vi "TEST - LVOOP Is Same Or Descendant Class.vi"(8 "error in (no error)":errorcluster) -> (0 "error out":errorcluster, 2 "Pass":bool)   [LabVIEW 2013]
uses:
  LVOOP Data/Class 2/Class 2.lvclass
  LVOOP Data/Class 3/Class 3.lvclass
  LVOOP Data/Class 1/Class 1.lvclass
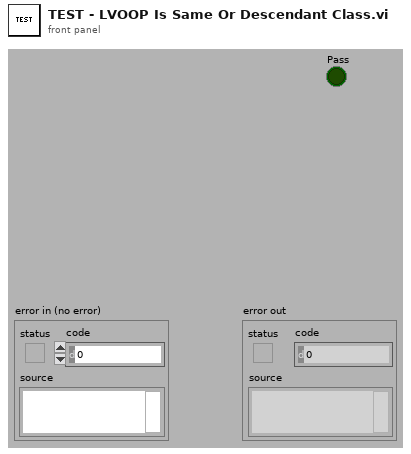
[diagram p1: front panel]
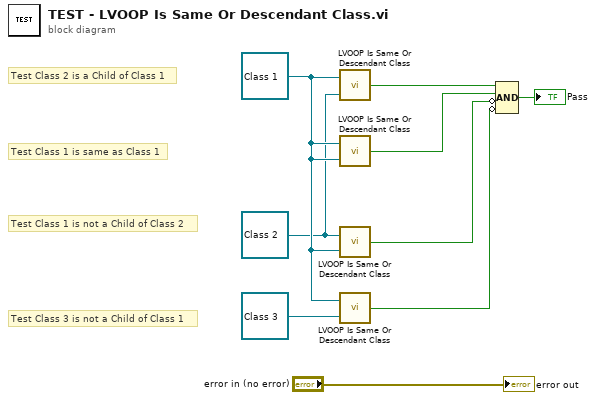
[diagram p0: block diagram]
diagram:
  w2 = refnum<class "Class 1.lvclass"> refnum ("Class 1.lvclass")
  w1 = refnum<class "Class 2.lvclass"> refnum ("Class 2.lvclass")
  # "Test Class 1 is same as Class 1"
  # "Test Class 1 is not a Child of Class 2"
  # "Test Class 3 is not a Child of Class 1"
  # "Test Class 2 is a Child of Class 1"
  n1 = call "LVOOP Is Same Or Descendant Class.vi"("Possible Descendant Object"=w1, "Object"=w2) -> ("Is Same Class or Descendant?"=w7:bool)
  n2 = call "LVOOP Is Same Or Descendant Class.vi"("Possible Descendant Object"=w2, "Object"=w2) -> ("Is Same Class or Descendant?"=w3:bool)
  n3 = call "LVOOP Is Same Or Descendant Class.vi"("Possible Descendant Object"=w2, "Object"=w1) -> ("Is Same Class or Descendant?"=w5:bool)
  n4 = call "LVOOP Is Same Or Descendant Class.vi"("Possible Descendant Object"=refnum<class "Class 3.lvclass"> refnum ("Class 3.lvclass"), "Object"=w2) -> ("Is Same Class or Descendant?"=w4:bool)
  n5 = Compound Arithmetic op=AND(w7, w3, invert w5, invert w4) -> (→"Pass":bool)
  "error out" <- "error in (no error)"
